vi "Validate JSON String.vi"(8 "error in (no error)":errorcluster, 11 "String":string) -> (0 "error out":errorcluster, 3 "session out":T1)   [LabVIEW 2017]
uses:
  <vilib>/userdefined/High Color/SLSC_Switch/nislscslSession.ctl
  <vilib>/SLSC_Switch/Get Topologies (Simulate).vi
  <vilib>/SLSC_Switch/Initialize with Topology (Simulate).vi
  <vilib>/SLSC_Switch/SLSC Switch.lvlib
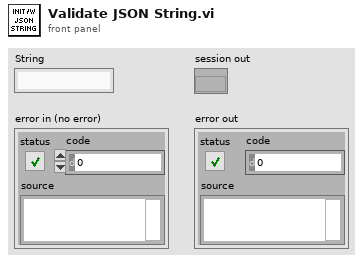
[diagram p1: front panel]
types:
  T1 = typedef "nislscslSession.ctl" = refnum<k20>
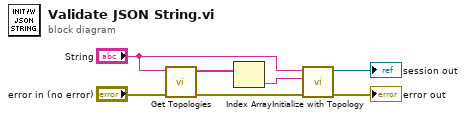
[diagram p0: block diagram]
diagram:
  n1 = call-poly <vilib>:"Get Topologies.vi"("error in (no error)"="error in (no error)", "switches json"="String") -> ("error out"=w7:errorcluster, "topologies"=w3:string[])  [unwired: 8 in]
  n2 = Index Array(array=w3) -> (element=w4:string)  [unwired: 1 in]
  n3 = call-poly <vilib>:"Initialize with Topology.vi"("error in (no error)"=w7, "topology"=w4, "switches json"="String") -> ("error out"=→"error out":errorcluster, "session out"=→"session out":T1)  [unwired: 7 in]
